vi "Experiment header-Save_Load config file data-retd.vi"(7 "Header file type":T7, 8 "error in (no error)":errorcluster, 9 "All header parameters in":T1={"Imaging Protocol"=enum."AOL Z-Stack", "Number of POI"=0, "Number of Miniscans"=0, "Number of Trials"=0, "Number of Cycles "=0, "# Averaged Frames"=0, "Laser power (%)"=0, "Pockels"=0.0, "Acquisition Length (sec)"=0.0, "Fill time (us)"=0.0, "POI Dwell time (us)"=0.0, "Miniscan Dwell time per pixel (us)"=0.0, "PMT 1"=0.0, "PMT 2"=0.0, "Back Apperture"=0.0, "Zoom"=0.0, "Frame Size"=200, "Center Frequency"=0.0, "Field of View"=0.0, "DwellTime (us)"=0.0, "Wavelength (nm)"=0.0, "AOL Z"=0.0, "AOL Mode"=enum."Raster", "GridXY"=0.0, "GridZ"=0.0, "TriggerDelay (sec)"=0.0, "Number of Pixels in Miniscan"=0, "Experiment folder path"=path "", "X centre"=0.0, "Y centre"=0.0, "Angle (degrees)"=0.0, "Plane Mode"=0, "Software version"=0.0, "Objective"="Olympus  20X", "MotorZ Calibration"=0, "Pockels Calibration"=0, "Threshold"=[], "Video length (sec)"=0.0, "Frame rate (fps)"=0, "Rectangle ROI length (pixels)"=0, "Rectangle ROI height (pixels)"=0} {"Pockels" format="%#.6g"; "Software version" format="%#.6g"; "Plane Mode" items=["XY Plane", "XZ Plane", "YZ Plane", "arbitraryplane"]; "Angle (degrees)" format="%#.6g"; "Frame Size" items=["100X100"=100, "128X128"=128, "200X200"=200, "256X256"=256, "512X512"=512, "1024x1024"=1024, "2048x2048"=2048]; "Back Apperture" format="%#.6g"; "PMT 2" format="%#.6g"; "PMT 1" format="%#.6g"; "Miniscan Dwell time per pixel (us)" format="%#.6g"; "Zoom" format="%#.6g"; "POI Dwell time (us)" format="%#.6g"; "Acquisition Length (sec)" format="%#.6g"; "Fill time (us)" format="%#.6g"}, 10 "Function":T8, 11 "Experiment data folder path":path) -> (0 "error out":errorcluster, 1 "All header parameters out":T1={"Imaging Protocol"=enum."AOL Z-Stack", "Number of POI"=0, "Number of Miniscans"=0, "Number of Trials"=0, "Number of Cycles "=0, "# Averaged Frames"=0, "Laser power (%)"=0, "Pockels"=0.0, "Acquisition Length (sec)"=0.0, "Fill time (us)"=0.0, "POI Dwell time (us)"=0.0, "Miniscan Dwell time per pixel (us)"=0.0, "PMT 1"=0.0, "PMT 2"=0.0, "Back Apperture"=0.0, "Zoom"=0.0, "Frame Size"=200, "Center Frequency"=0.0, "Field of View"=0.0, "DwellTime (us)"=0.0, "Wavelength (nm)"=0.0, "AOL Z"=0.0, "AOL Mode"=enum."Raster", "GridXY"=0.0, "GridZ"=0.0, "TriggerDelay (sec)"=0.0, "Number of Pixels in Miniscan"=0, "Experiment folder path"=path "", "X centre"=0.0, "Y centre"=0.0, "Angle (degrees)"=0.0, "Plane Mode"=0, "Software version"=0.0, "Objective"="Olympus  20X", "MotorZ Calibration"=0, "Pockels Calibration"=0, "Threshold"=[], "Video length (sec)"=0.0, "Frame rate (fps)"=0, "Rectangle ROI length (pixels)"=0, "Rectangle ROI height (pixels)"=0} {"Pockels" format="%#.6g"; "Software version" format="%#.6g"; "Plane Mode" items=["XY Plane", "XZ Plane", "YZ Plane", "arbitraryplane"]; "Angle (degrees)" format="%#.6g"; "Frame Size" items=["100X100"=100, "128X128"=128, "200X200"=200, "256X256"=256, "512X512"=512, "1024x1024"=1024, "2048x2048"=2048]; "Back Apperture" format="%#.6g"; "PMT 2" format="%#.6g"; "PMT 1" format="%#.6g"; "Miniscan Dwell time per pixel (us)" format="%#.6g"; "Zoom" format="%#.6g"; "POI Dwell time (us)" format="%#.6g"; "Acquisition Length (sec)" format="%#.6g"; "Fill time (us)" format="%#.6g"})   [LabVIEW 2017]
doc: "This self-contained module handles all header files save/write operations.\nIt can generate a number of different header files containing different parameters.\nEach different type of header file has its own type defined cluster of parameters.\nThe functionality is fully self-scalable such as when new parameters are added or parameters are deleted or renamed in the typedef clusters this is all handled automatically without the need for further updates to this module."
uses:
  Typedefs/Header parameters cluster-ALL-retd.ctl
  Typedefs/Imaging Protocols enum.ctl
  Typedefs/Frame Size.ctl
  Typedefs/AOL modes.ctl
  Typedefs/Plane Mode.ctl
  Typedefs/Objective selector control enum.ctl
  Typedefs/Save-Load-Save as-Load last enum.ctl
  Typedefs/Header file type enum.ctl
  <vilib>/Utility/config.llb/Read Key (Double).vi
  <vilib>/Utility/config.llb/Write Key (Double).vi
  <vilib>/Utility/config.llb/NI_LVConfig.lvlib
panel:
  # "Actual FOV ------>\n(not norm FOFV)"
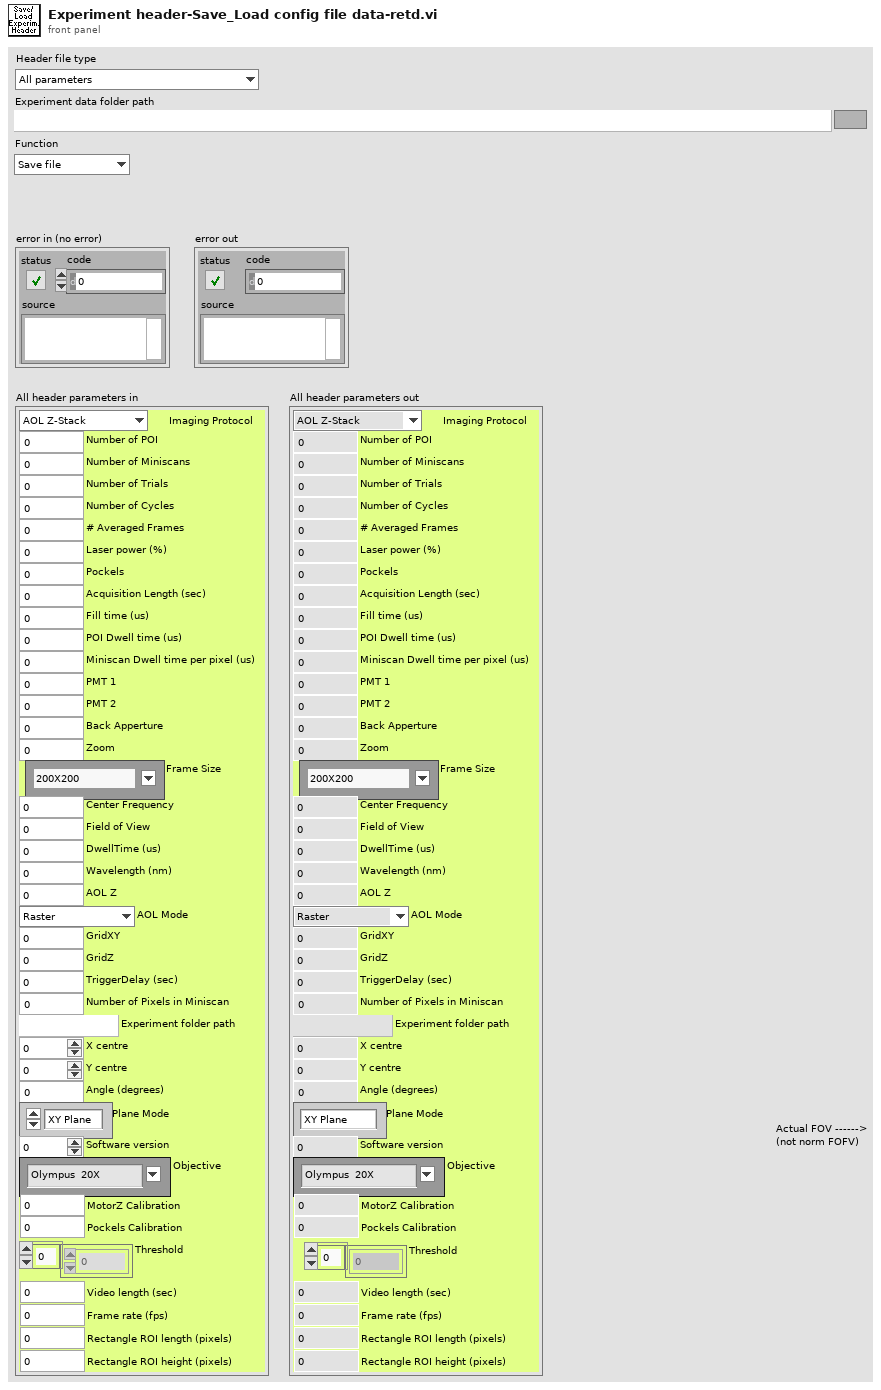
[diagram p1: front panel]
types:
  T1 = typedef "Header parameters cluster-ALL-retd.ctl" = cluster{"Imaging Protocol":T2, "Number of POI":u16, "Number of Miniscans":u16, "Number of Trials":u16, "Number of Cycles ":u64, "# Averaged Frames":u16, "Laser power (%)":u8, "Pockels":dbl, "Acquisition Length (sec)":dbl, "Fill time (us)":dbl, "POI Dwell time (us)":dbl, "Miniscan Dwell time per pixel (us)":dbl, "PMT 1":dbl, "PMT 2":dbl, "Back Apperture":dbl, "Zoom":dbl, "Frame Size":T3, "Center Frequency":dbl, "Field of View":dbl, "DwellTime (us)":dbl, "Wavelength (nm)":dbl, "AOL Z":dbl, "AOL Mode":T4, "GridXY":dbl, "GridZ":dbl, "TriggerDelay (sec)":dbl, "Number of Pixels in Miniscan":u16, "Experiment folder path":path, "X centre":dbl, "Y centre":dbl, "Angle (degrees)":dbl, "Plane Mode":T5, "Software version":dbl, "Objective":T6, "MotorZ Calibration":u32, "Pockels Calibration":u32, "Threshold":u16[], "Video length (sec)":dbl, "Frame rate (fps)":u8, "Rectangle ROI length (pixels)":u16, "Rectangle ROI height (pixels)":u16}
  T2 = typedef "Imaging Protocols enum.ctl" = enum16{"AOL Z-Stack", "Motor Z Stack", "Functional Acquisition", "Single Plane Acquisition", "Volume Acquisition", "Live Imaging", "Live Plane Imaging", "Live Volume Imaging"}
  T3 = typedef "Frame Size.ctl" = u16
  T4 = typedef "AOL modes.ctl" = enum16{"Raster", "Structural", "Pointing", "Mini Scan", "Alignment"}
  T5 = typedef "Plane Mode.ctl" = u16
  T6 = typedef "Objective selector control enum.ctl" = string
  T7 = typedef "Header file type enum.ctl" = enum16{"All parameters", "Login", "Global Parameters", "Imaging Modes", "Time Series", "Motor Zstack", "AOL Zstack", "Functional Imaging", "Movement Correction", "Calibration Setup", "Statistics", "Biology Information"}
  T8 = typedef "Save-Load-Save as-Load last enum.ctl" = enum16{"Save file", "Save file as", "Load file", "Load last file"}
  T9 = typedef "Fixed strings.ctl" = cluster{"ROI file name":string, "Normalised ROI file name":string, "Zplane Pockels values file name":string, "Functional data folder name":string, "Experiment Header file name":string, "Z-stack images folder name":string, "Groups setup rel. path":string, "Groups text file rel. path":string, "TDMS files folder name (F.img)":string, "TDMS files folder name (V.acq)":string, "TDMS files folder name (Pl.acq)":string, "Cycle rel times sequence file":string, "Dynamically called VIs folder name":string, "Time Series folder base name":string}
  T10 = typedef "NI_LVConfig.lvlib/Config Data RefNum.ctl" = refnum<k1>
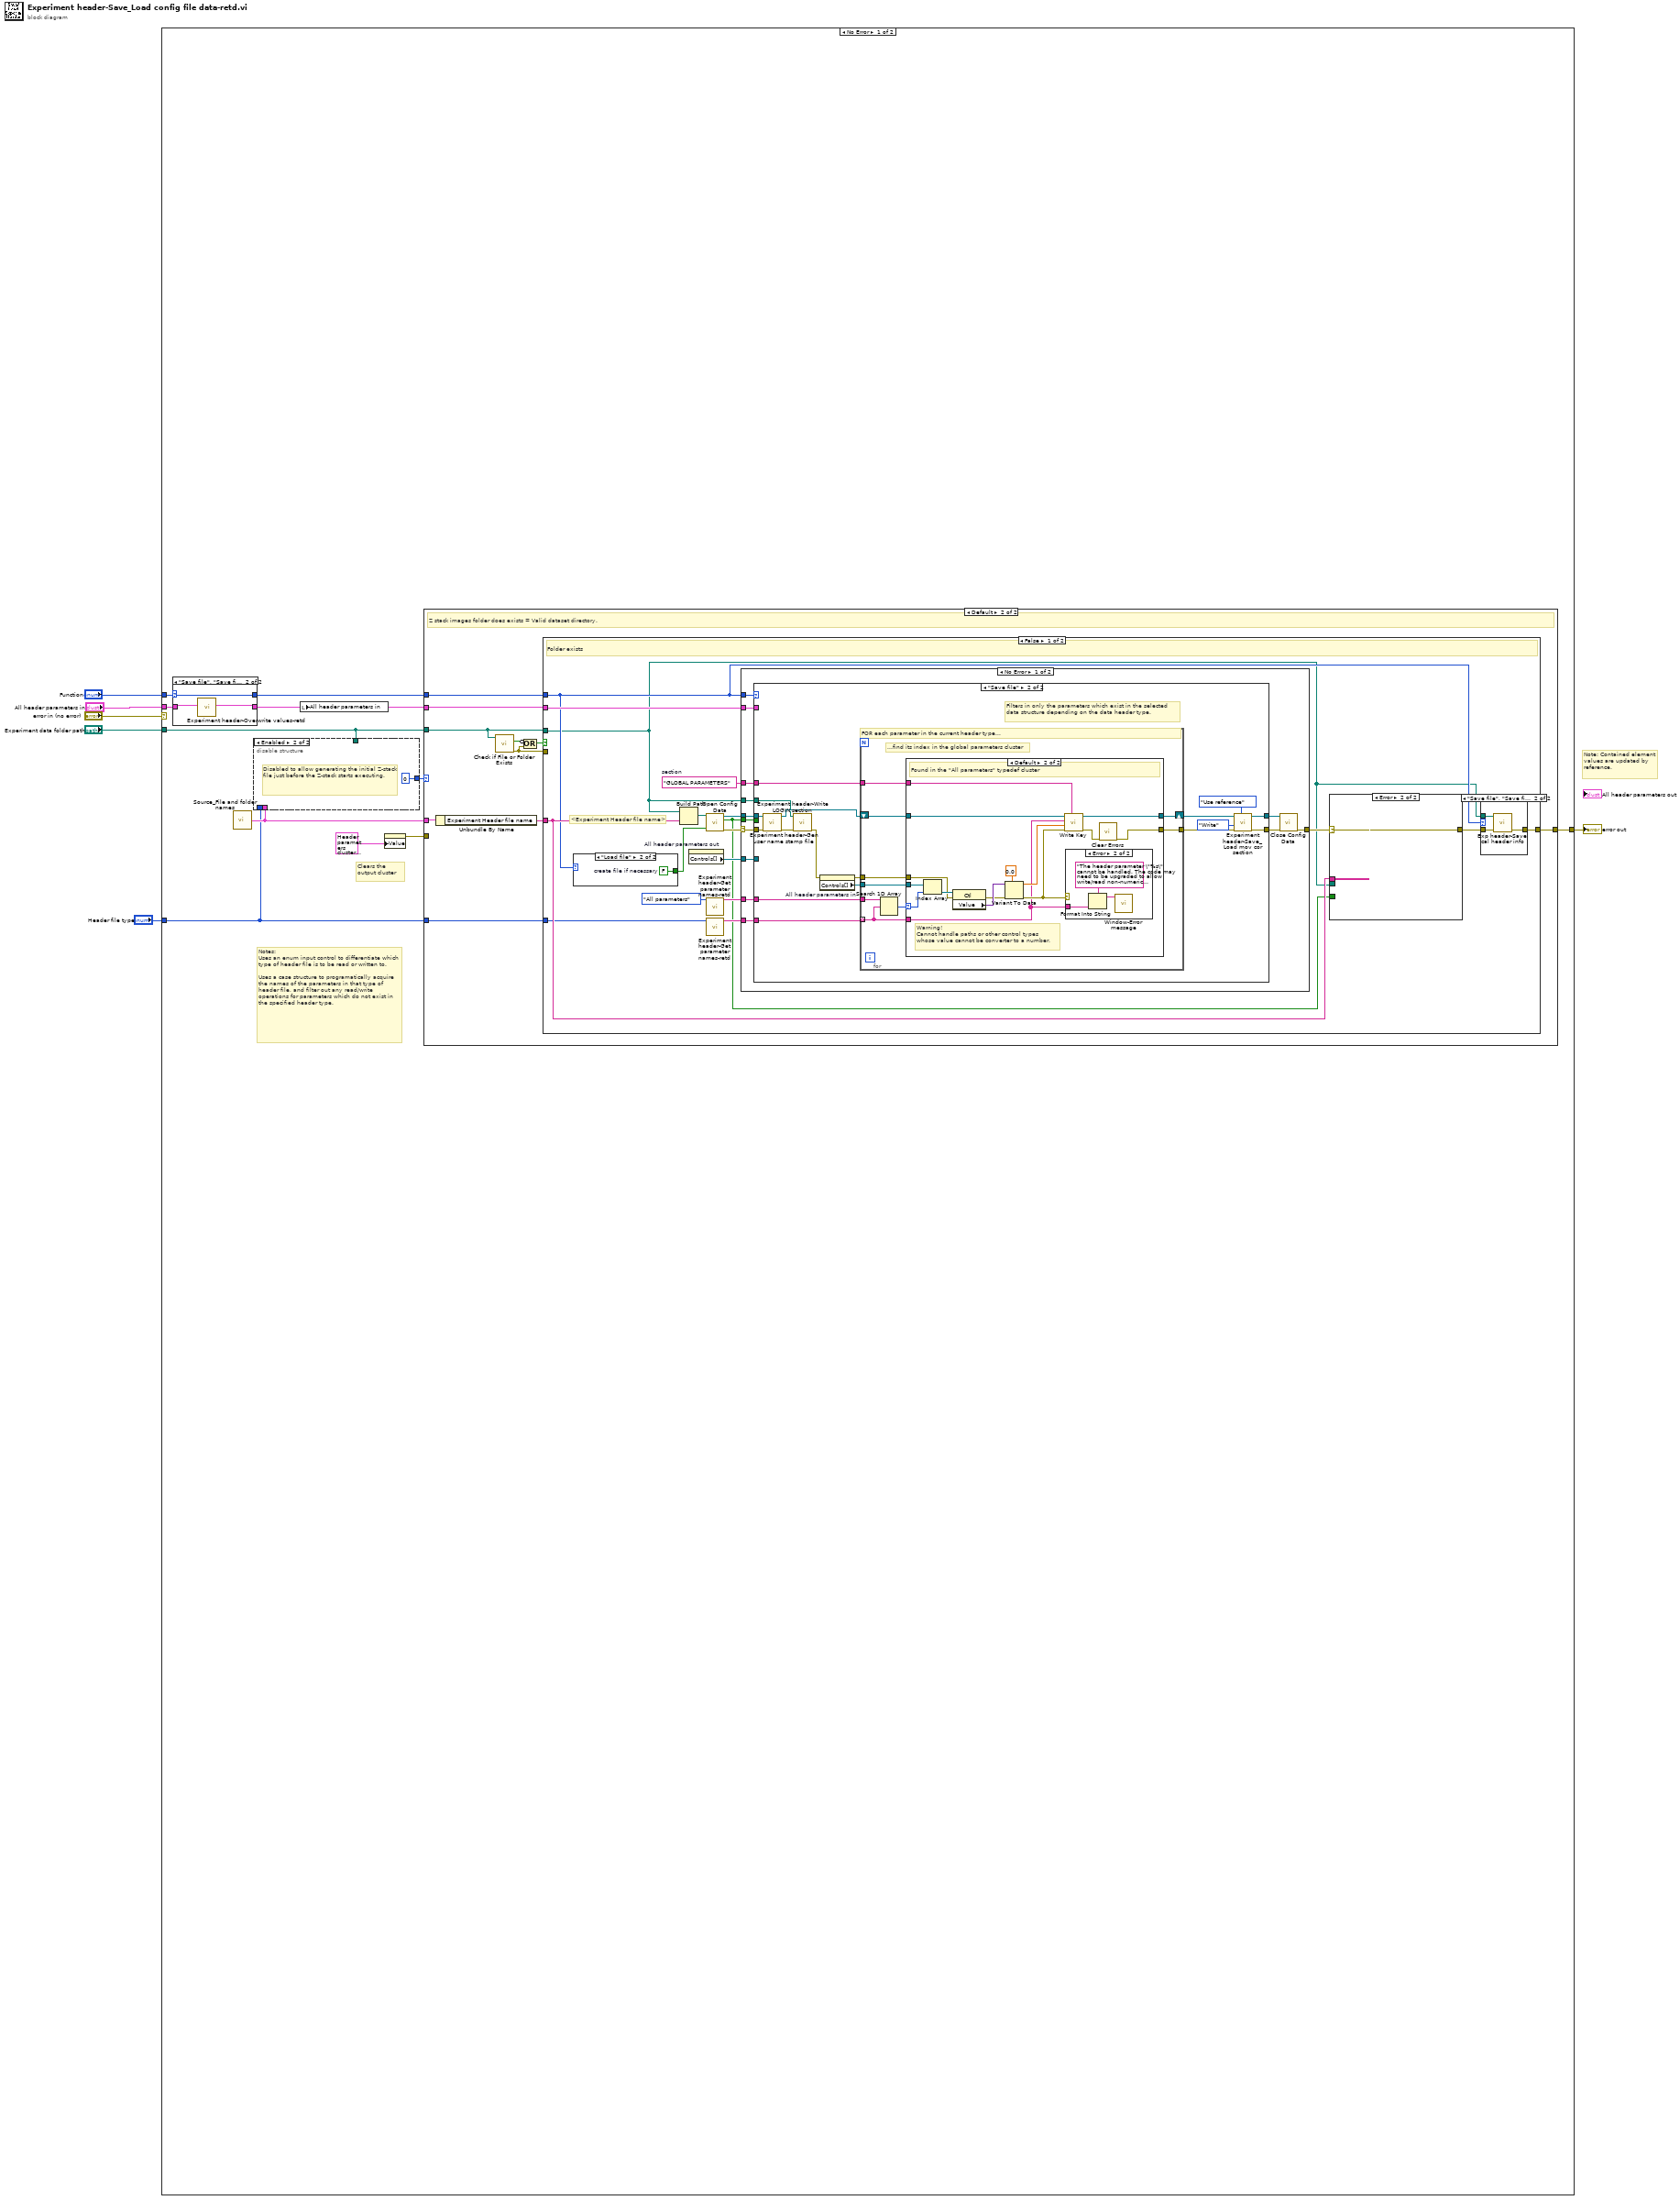
[diagram p0: block diagram]
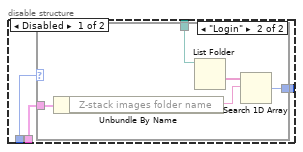
[diagram p3: hidden frame]
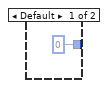
[diagram p4: hidden frame]
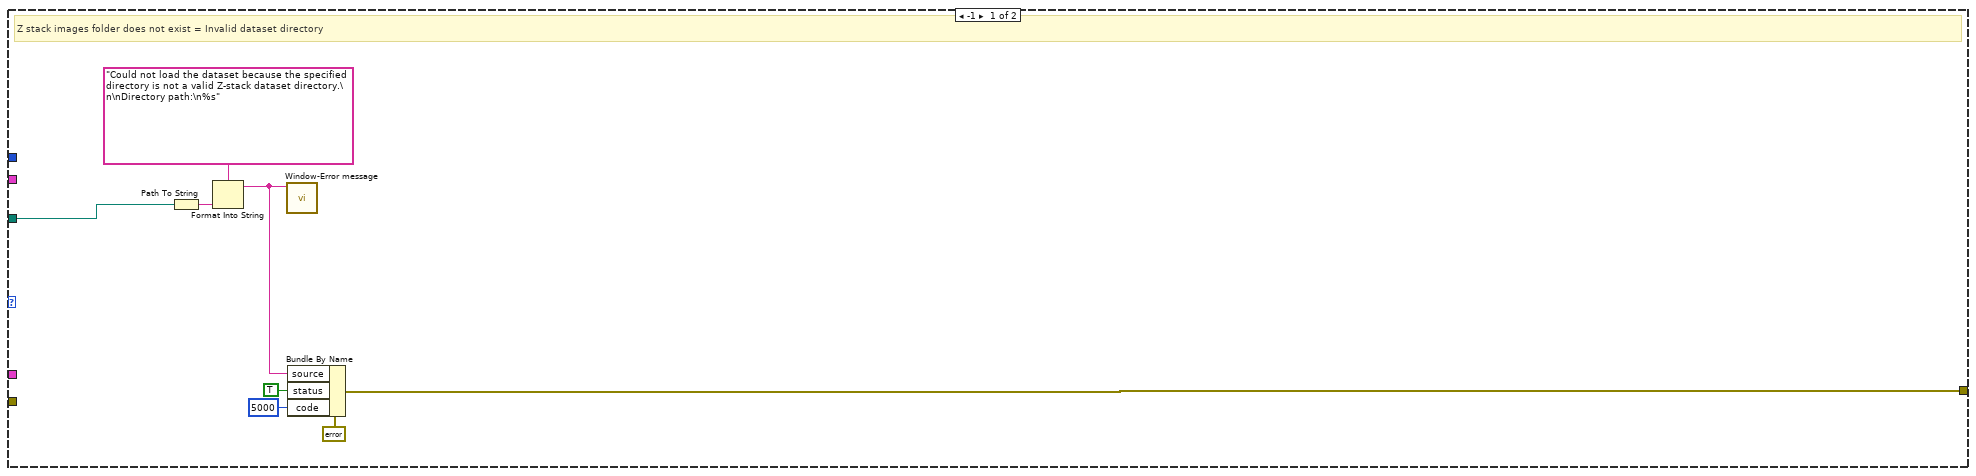
[diagram p5: hidden frame]
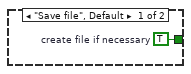
[diagram p7: hidden frame]
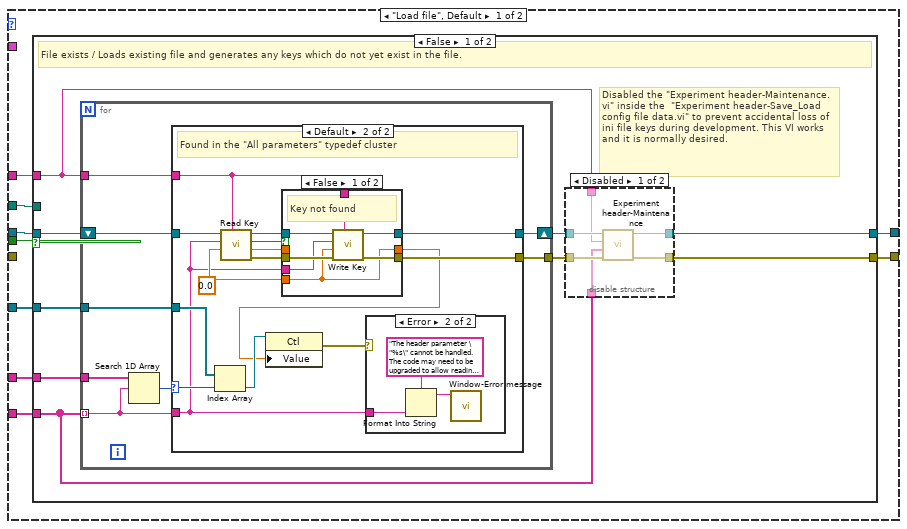
[diagram p8: hidden frame]
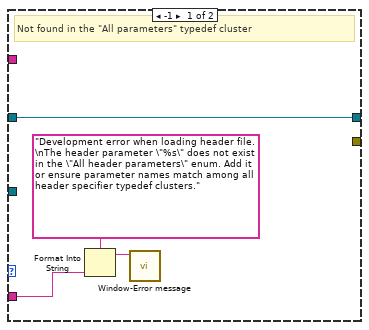
[diagram p10: hidden frame]
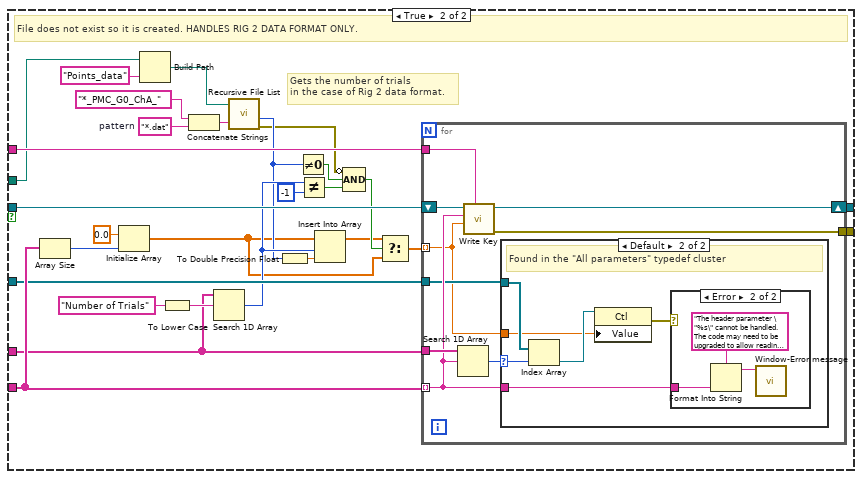
[diagram p13: hidden frame]
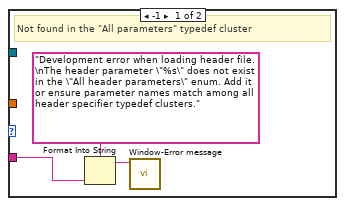
[diagram p14: hidden frame]
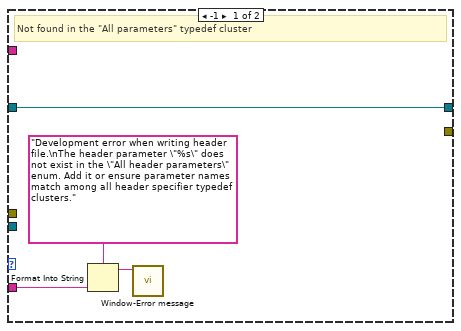
[diagram p16: hidden frame]
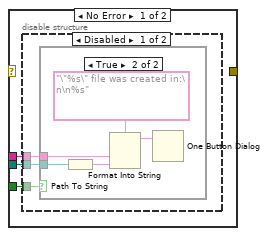
[diagram p19: hidden frame]
diagram:
  # "Note: Contained element values are updated by reference."
  n1 = case shown="No Error" "error in (no error)" {
    selector: "error in (no error)" -> [_ w277]
    tunnel: [w17 w277] -> w6
    tunnel: "Function" -> [w11 _]
    tunnel: "Experiment data folder path" -> [w9 _]
    tunnel: "Header file type" -> [w13 _]
    tunnel: "All header parameters in" -> [w10 _]
    frame No Error {
      # "Clears the output cluster"
      # "Notes:\nUses an enum input control to differentiate which type of header file is to be read or written to.\n\nUses a case structure to programatically acquire the names of the parameters in that type of header file, and filter out any read/write operations for parameters which do not exist in the specified header type."
      n2 = case shown="\"Save file\", \"Save file as\"" w11 {
        selector: w11 -> [w19 w22]
        tunnel: [w18 w20] -> w8
        tunnel: [w19 w22] -> w12
        tunnel: w10 -> [w18 w21]
        frame Default {
        }
        frame "Save file", "Save file as" {
          n3 = call "Experiment header-Overwrite values-retd.vi"("All header parameters in"=w21) -> ("All header parameters (FOV converted to um)"=w20:T1)  [unwired: 9 in, 1 out]
        }
      }
      n4 = call "Source_File and folder names.vi"() -> ("Fixed strings"=w15:T9)  [unwired: 1 in]
      n5 = disable-structure shown="Enabled" {
        disable-tunnel: w9 -> [w26 _]
        disable-tunnel: [w25 0 ("index of element")] -> w16
        disable-tunnel: w15 -> [w24 _]
        disable-tunnel: w13 -> [w23 _]
        frame Disabled {
          n6 = case shown="\"Login\"" w23 {
            tunnel: w26 -> [_ w31]
            tunnel: [0 ("index of element") w30] -> w25
            tunnel: w24 -> [_ w28]
            frame Default {
            }
            frame "Login" {
              n7 = Unbundle By Name(w28) -> ("Z-stack images folder name"=w29:string)
              n8 = List Folder(path=w31) -> (folder names=w32:string[])  [unwired: 3 in, 3 out]
              n9 = Search 1D Array(1D array=w32, element=w29) -> (index of element=w30:i32)  [unwired: 1 in]
            }
          }
        }
        frame Enabled {
          # "Disabled to allow generating the initial Z-stack file just before the Z-stack starts executing."
        }
      }
      n10 = local write "All header parameters in"(w8) -> ()
      n11 = property on="All header parameters out" class="Clust (strict)"("Value"=T1 {"Imaging Protocol"=enum."AOL Z-Stack", "Number of POI"=0, "Number of Miniscans"=0, "Number of Trials"=0, "Number of Cycles "=0, "# Averaged Frames"=0, "Laser power (%)"=0, "Pockels"=0.0, "Acquisition Length (sec)"=0.0, "Fill time (us)"=0.0, "POI Dwell time (us)"=0.0, "Miniscan Dwell time per pixel (us)"=0.0, "PMT 1"=0.0, "PMT 2"=0.0, "Back Apperture"=0.0, "Zoom"=0.0, "Frame Size"=200, "Center Frequency"=0.0, "Field of View"=0.0, "DwellTime (us)"=0.0, "Wavelength (nm)"=0.0, "AOL Z"=0.0, "AOL Mode"=enum."Raster", "GridXY"=0.0, "GridZ"=0.0, "TriggerDelay (sec)"=0.0, "Number of Pixels in Miniscan"=0, "Experiment folder path"=path "", "X centre"=0.0, "Y centre"=0.0, "Angle (degrees)"=0.0, "Plane Mode"=0, "Software version"=0.0, "Objective"="Olympus  20X", "MotorZ Calibration"=0, "Pockels Calibration"=0, "Threshold"=[], "Video length (sec)"=0.0, "Frame rate (fps)"=0, "Rectangle ROI length (pixels)"=0, "Rectangle ROI height (pixels)"=0} ("All header parameters / Header module interface cluster")) -> (error out=w14:errorcluster)  [unwired: 2 in, 1 out]
      n12 = case shown="Default" w16 {
        tunnel: [w34 w51] -> w17
        tunnel: w12 -> [_ w47]
        tunnel: w8 -> [_ w46]
        tunnel: w9 -> [w39 w45]
        tunnel: w15 -> [_ w43]
        tunnel: w13 -> [_ w42]
        tunnel: w14 -> [_ _]
        frame -1 {
          # "Z stack images folder does not exist = Invalid dataset directory"
          n13 = Path To String(path=w39) -> (string=w41:string)
          n14 = Format Into String(format string="Could not load the dataset because the specified directory is not a valid Z-stack dataset directory.\n\nDirectory path:\n%s" ("message"), w41) -> (resulting string=w35:string)  [unwired: 2 in, 1 out]
          n15 = call "Window-Error message.vi"("Message"=w35) -> ()  [unwired: 10 in, 1 out]
          n16 = Bundle By Name(cluster=errorcluster {"status"=FALSE, "code"=0, "source"=""} ("error out"), "source"=w35, "status"=TRUE, "code"=5000) -> (w34:errorcluster)
        }
        frame Default {
          # "Z stack images folder does exists = Valid dataset directory."
          n17 = Unbundle By Name(w43) -> ("Experiment Header file name"=w44:string)
          n18 = call <vilib>:"Check if File or Folder Exists.vi"("path"=w45) -> ("error out"=w48:errorcluster, "file or folder exists?"=w50:bool)  [unwired: 8 in, 1 out]
          n19 = Compound Arithmetic op=OR(invert w50, w48) -> (w49:bool)
          n20 = case shown="False" w49 {
            tunnel: [w55 w266] -> w51
            tunnel: w44 -> [w64 _]
            tunnel: w45 -> [w52 w267]
            tunnel: w48 -> [_ w265]
            tunnel: w47 -> [w53 _]
            tunnel: w46 -> [w69 _]
            tunnel: w42 -> [w63 _]
            frame False {
              w58 = "GLOBAL PARAMETERS"  # section
              # "<Experiment Header file name>"
              # "Folder exists"
              n21 = case shown="\"Load file\"" w53 {
                tunnel: [w74 w75] -> w56
                frame "Save file", Default {
                  w74 = TRUE  # create file if necessary
                }
                frame "Load file" {
                  w75 = FALSE  # create file if necessary
                }
              }
              n22 = Build Path(base path=w52, name or relative path=w64) -> (appended path=w68:path)
              n23 = property on="All header parameters out" class="Clust (strict)"() -> ("Controls[]"=w60:refnum<vi>[])  [unwired: 2 in, 2 out]
              n24 = call <vilib>:"Open Config Data.vi"("create file if necessary (T)"=w56, "configuration file path"=w68) -> ("error out"=w61:errorcluster, "file created?"=w59:bool, "refnum"=w67:T10)  [unwired: 7 in]
              n25 = call "Experiment header-Get parameter names-retd.vi"("Header file type"=Header_file_type_enum."All parameters") -> ("Parameter names"=w62:string[])  [unwired: 9 in, 1 out]
              n26 = call "Experiment header-Get parameter names-retd.vi"("Header file type"=w63) -> ("Parameter names"=w65:string[])  [unwired: 9 in, 1 out]
              n27 = case shown="No Error" w61 {
                selector: w61 -> [w76 w252]
                tunnel: w58 -> [w88 _]
                tunnel: w53 -> [w87 _]
                tunnel: w69 -> [w86 _]
                tunnel: w67 -> [w85 _]
                tunnel: [w82 w252] -> w66
                tunnel: w65 -> [w81 _]
                tunnel: w52 -> [w80 _]
                tunnel: w59 -> [w79 _]
                tunnel: w62 -> [w78 _]
                tunnel: w60 -> [w77 _]
                frame No Error {
                  n28 = case shown="\"Save file\"" w87 {
                    tunnel: [w92 w214] -> w83
                    tunnel: w88 -> [w97 w220]
                    tunnel: w86 -> [_ _]
                    tunnel: w81 -> [w96 w219]
                    tunnel: w79 -> [w94 _]
                    tunnel: w85 -> [w95 w218]
                    tunnel: [w93 w212] -> w84
                    tunnel: w80 -> [w91 w206]
                    tunnel: w78 -> [w90 w217]
                    tunnel: w77 -> [w89 _]
                    tunnel: w76 -> [_ w208]
                    frame "Load file", Default {
                      n29 = case shown="False" w94 {
                        tunnel: w95 -> [w106 w182]
                        tunnel: w97 -> [w99 w181]
                        tunnel: w96 -> [w100 w170]
                        tunnel: [w103 w180] -> w93
                        tunnel: [w102 w179] -> w92
                        tunnel: w91 -> [_ w169]
                        tunnel: w90 -> [w101 w166]
                        tunnel: w89 -> [w98 w165]
                        frame False {
                          # "Disabled the \"Experiment header-Maintenance.vi\" inside the  \"Experiment header-Save_Load config file data.vi\" to prevent accidental loss of ini file keys during development. This VI works and it is normally desired."
                          # "File exists / Loads existing file and generates any keys which do not yet exist in the file."
                          n30 = for {
                            shift-right: [w121] -> w105
                            shift-left: w106 -> [w122]
                            tunnel: w99 -> [w120]
                            tunnel: [w119] -> w104
                            tunnel: w100 -> [w117] mode=indexing
                            tunnel: w101 -> [w118]
                            tunnel: w98 -> [w115]
                            n31 = Search 1D Array(1D array=w118, element=w117) -> (index of element=w116:i32)  [unwired: 1 in]
                            n32 = case shown="Default" w116 {
                              selector: w116 -> [_ w131]
                              tunnel: w122 -> [w124 w141]
                              tunnel: [w124 w139] -> w121
                              tunnel: w120 -> [_ w137]
                              tunnel: [_ w135] -> w119
                              tunnel: w117 -> [w123 w127]
                              tunnel: w115 -> [_ w130]
                              frame -1 {
                                # "Not found in the \"All parameters\" typedef cluster"
                                n33 = Format Into String(format string="Development error when loading header file.\nThe header parameter \"%s\" does not exist in the \"All header parameters\" enum. Add it or ensure parameter names match among all header specifier typedef clusters.", w123) -> (resulting string=w125:string)  [unwired: 2 in, 1 out]
                                n34 = call "Window-Error message.vi"("Message"=w125) -> ()  [unwired: 10 in, 1 out]
                              }
                              frame Default {
                                w133 = 0.0 ("default value")
                                # "Found in the \"All parameters\" typedef cluster"
                                n35 = Index Array(array=w130, index=w131) -> (element=w132:refnum<vi>)
                                n36 = call-poly <vilib>:"Read Key.vi"("section"=w137, "default value"=w133, "key"=w127, "refnum"=w141) -> ("error out"=w136:errorcluster, "value"=w138:dbl, "found?"=w134:bool, "refnum out"=w140:T10)  [unwired: 4 in]
                                n37 = case shown="False" w134 {
                                tunnel: w140 -> [w151 w154]
                                tunnel: [w150 w154] -> w139
                                tunnel: w138 -> [_ w153]
                                tunnel: [w146 w153] -> w129
                                tunnel: w137 -> [w149 _]
                                tunnel: w133 -> [w146 _]
                                tunnel: w136 -> [w148 w152]
                                tunnel: [w147 w152] -> w135
                                tunnel: w127 -> [w145 _]
                                frame False {
                                # "Key not found"
                                n38 = call-poly <vilib>:"Write Key.vi"("section"=w149, "error in (no error)"=w148, "value"=w146, "key"=w145, "refnum"=w151) -> ("error out"=w147:errorcluster, "refnum out"=w150:T10)  [unwired: 4 in, 1 out]
                                }
                                frame True {
                                # "Key found"
                                }
                                }
                                n39 = property class="Ctl"(reference=w132, "Value"=w129) -> (error out=w128:errorcluster)  [unwired: 1 in, 1 out]
                                n40 = case shown="Error" w128 {
                                tunnel: w127 -> [_ w143]
                                frame No Error {
                                }
                                frame Error {
                                n41 = Format Into String(format string="The header parameter \"%s\" cannot be handled. The code may need to be upgraded to allow reading non-numeric parameter values from the header file.", w143) -> (resulting string=w144:string)  [unwired: 2 in, 1 out]
                                n42 = call "Window-Error message.vi"("Message"=w144) -> ()  [unwired: 10 in, 1 out]
                                }
                                }
                              }
                            }
                          }
                          n43 = disable-structure shown="Disabled" {
                            disable-tunnel: w105 -> [w112 w114]
                            disable-tunnel: w104 -> [w111 w113]
                            disable-tunnel: [w110 w114] -> w103
                            disable-tunnel: [w109 w113] -> w102
                            disable-tunnel: w100 -> [w108 _]
                            disable-tunnel: w99 -> [w107 _]
                            frame Disabled {
                              n44 = call "Experiment header-Maintenance.vi"("error in (no error)"=w111, "<Valid parameter names>"=w108, "section"=w107, "Experiment header file ref in"=w112) -> ("error out"=w109:errorcluster, "Experiment header file ref"=w110:T10)  [unwired: 6 in]
                            }
                            frame Enabled {
                            }
                          }
                        }
                        frame True {
                          w175 = "*.dat"  # pattern
                          # "Gets the number of trials\nin the case of Rig 2 data format."
                          # "File does not exist so it is created. HANDLES RIG 2 DATA FORMAT ONLY."
                          n45 = Array Size(array=w170) -> (size(s)=w173:i32)
                          n46 = Initialize Array(0.0, w173) -> (w157:dbl[])
                          n47 = Build Path(base path=w169, name or relative path="Points_data") -> (appended path=w174:path)
                          n48 = To Lower Case(string="Number of Trials" ("element")) -> (all lower case string=w167:string)
                          n49 = Concatenate Strings("*_PMC_G0_ChA_" ("string"), w175) -> (w176:string)
                          n50 = Search 1D Array(1D array=w166, element=w167) -> (index of element=w164:i32)  [unwired: 1 in]
                          n51 = call <vilib>:"Recursive File List.vi"("pattern"=w176, "Folder Path"=w174) -> ("error out"=w155:errorcluster, "Number of Files"=w162:i32)  [unwired: 5 in, 3 out]
                          n52 = To Double Precision Float(number=w162) -> (double precision float=w171:dbl)
                          n53 = Not Equal To 0?(x=w162) -> (x != 0?=w161:bool)
                          n54 = Not Equal?(x=w164, y=-1) -> (x != y?=w160:bool)
                          n55 = Insert Into Array(array=w157, index=w164, new element=w171) -> (w158:dbl[])
                          n56 = Compound Arithmetic op=AND(invert w155, w161, w160) -> (w159:bool)
                          n57 = Select(t=w158, s=w159, f=w157) -> (s? t:f=w156:dbl[])
                          n58 = for {
                            shift-right: [w190] -> w180
                            shift-left: w182 -> [w191]
                            tunnel: w181 -> [w189]
                            tunnel: [w188] -> w179
                            tunnel: w170 -> [w185] mode=indexing
                            tunnel: w156 -> [w183] mode=indexing
                            tunnel: w166 -> [w186]
                            tunnel: w165 -> [w184]
                            n59 = Search 1D Array(1D array=w186, element=w185) -> (index of element=w187:i32)  [unwired: 1 in]
                            n60 = call-poly <vilib>:"Write Key.vi"("section"=w189, "value"=w183, "key"=w185, "refnum"=w191) -> ("error out"=w188:errorcluster, "refnum out"=w190:T10)  [unwired: 5 in, 1 out]
                            n61 = case shown="Default" w187 {
                              selector: w187 -> [_ w199]
                              tunnel: w185 -> [w192 w196]
                              tunnel: w184 -> [_ w198]
                              tunnel: w183 -> [_ w195]
                              frame -1 {
                                # "Not found in the \"All parameters\" typedef cluster"
                                n62 = Format Into String(format string="Development error when loading header file.\nThe header parameter \"%s\" does not exist in the \"All header parameters\" enum. Add it or ensure parameter names match among all header specifier typedef clusters.", w192) -> (resulting string=w193:string)  [unwired: 2 in, 1 out]
                                n63 = call "Window-Error message.vi"("Message"=w193) -> ()  [unwired: 10 in, 1 out]
                              }
                              frame Default {
                                # "Found in the \"All parameters\" typedef cluster"
                                n64 = Index Array(array=w198, index=w199) -> (element=w200:refnum<vi>)
                                n65 = property class="Ctl"(reference=w200, "Value"=w195) -> (error out=w197:errorcluster)  [unwired: 1 in, 1 out]
                                n66 = case shown="Error" w197 {
                                tunnel: w196 -> [_ w202]
                                frame No Error {
                                }
                                frame Error {
                                n67 = Format Into String(format string="The header parameter \"%s\" cannot be handled. The code may need to be upgraded to allow reading non-numeric parameter values from the header file.", w202) -> (resulting string=w203:string)  [unwired: 2 in, 1 out]
                                n68 = call "Window-Error message.vi"("Message"=w203) -> ()  [unwired: 10 in, 1 out]
                                }
                                }
                              }
                            }
                          }
                        }
                      }
                    }
                    frame "Save file" {
                      # "Filters in only the parameters which exist in the selected data structure depending on the data header type."
                      n69 = call "Experiment header-Write LOGIN section.vi"("error in (no error)"=w208, "Experiment header file ref"=w218) -> ("error out"=w205:errorcluster, "Experiment header file ref"=w209:T10)  [unwired: 8 in]
                      n70 = call "Experiment header-Gen user name stamp file.vi"("error in (no error)"=w205, "Experiment data folder path"=w206) -> ("error out"=w204:errorcluster)  [unwired: 9 in]
                      n71 = property on="All header parameters in" class="Clust (strict)"(error in=w204) -> (error out=w207:errorcluster, "Controls[]"=w216:refnum<vi>[])  [unwired: 1 in, 1 out]
                      n72 = for {
                        shift-right: [w228] -> w215
                        shift-left: w209 -> [w229]
                        tunnel: w220 -> [w227]
                        tunnel: w219 -> [w224] mode=indexing
                        tunnel: w217 -> [w225]
                        tunnel: w216 -> [w223]
                        tunnel: [w222] -> w213
                        tunnel: w207 -> [w221]
                        # "...find its index in the global parameters cluster"
                        # "FOR each parameter in the current header type..."
                        n73 = Search 1D Array(1D array=w225, element=w224) -> (index of element=w226:i32)  [unwired: 1 in]
                        n74 = case shown="Default" w226 {
                          selector: w226 -> [_ w245]
                          tunnel: w229 -> [w233 w248]
                          tunnel: [w233 w247] -> w228
                          tunnel: w227 -> [_ w246]
                          tunnel: w224 -> [w232 w237]
                          tunnel: w223 -> [_ w241]
                          tunnel: [_ w235] -> w222
                          tunnel: w221 -> [_ w234]
                          frame -1 {
                            # "Not found in the \"All parameters\" typedef cluster"
                            n75 = Format Into String(format string="Development error when writing header file.\nThe header parameter \"%s\" does not exist in the \"All header parameters\" enum. Add it or ensure parameter names match among all header specifier typedef clusters.", w232) -> (resulting string=w231:string)  [unwired: 2 in, 1 out]
                            n76 = call "Window-Error message.vi"("Message"=w231) -> ()  [unwired: 10 in, 1 out]
                          }
                          frame Default {
                            # "Warning!\nCannot handle paths or other control types \nwhose value cannot be converter to a number."
                            # "Found in the \"All parameters\" typedef cluster"
                            n77 = Index Array(array=w241, index=w245) -> (element=w244:refnum<vi>)
                            n78 = property class="Ctl"(reference=w244, error in=w234) -> (error out=w239:errorcluster, "Value"=w243:variant)  [unwired: 1 out]
                            n79 = Variant To Data(error in=w239, type=0.0, Variant=w243) -> (data=w240:dbl, error out=w238:errorcluster)
                            n80 = call-poly <vilib>:"Write Key.vi"("section"=w246, "error in (no error)"=w238, "value"=w240, "key"=w237, "refnum"=w248) -> ("error out"=w236:errorcluster, "refnum out"=w247:T10)  [unwired: 4 in, 1 out]
                            n81 = case shown="Error" w238 {
                              tunnel: w237 -> [_ w249]
                              frame No Error {
                              }
                              frame Error {
                                n82 = Format Into String(format string="The header parameter \"%s\" cannot be handled. The code may need to be upgraded to allow write/read non-numeric parameter values to the header file.", w249) -> (resulting string=w250:string)  [unwired: 2 in, 1 out]
                                n83 = call "Window-Error message.vi"("Message"=w250) -> ()  [unwired: 10 in, 1 out]
                              }
                            }
                            n84 = call <vilib>:"Clear Errors.vi"("error in (no error)"=w236) -> ("error out"=w235:errorcluster)  [unwired: 5 in, 1 out]
                          }
                        }
                      }
                      n85 = call "Experiment header-Save_Load mov cor section.vi"("Input Mode (ref)"=enum16{"Use reference", "Use folder path"}."Use reference", "error in (no error)"=w213, "Function"=enum16{"Write", "Read"}."Write", "Exp header file ref in"=w215) -> ("error out"=w214:errorcluster, "Exp header file ref"=w212:T10)  [unwired: 5 in, 1 out]
                    }
                  }
                  n86 = call <vilib>:"Close Config Data.vi"("error in (no error)"=w83, "refnum"=w84) -> ("error out"=w82:errorcluster)  [unwired: 8 in, 1 out]
                }
                frame Error {
                }
              }
              n87 = case shown="Error" w66 {
                selector: w66 -> [_ w264]
                tunnel: [_ w264] -> w54
                tunnel: w59 -> [w255 _]
                tunnel: w52 -> [w254 _]
                tunnel: w64 -> [w253 _]
                frame No Error {
                  n88 = disable-structure shown="Disabled" {
                    disable-tunnel: w255 -> [w258 _]
                    disable-tunnel: w254 -> [w257 _]
                    disable-tunnel: w253 -> [w256 _]
                    frame Disabled {
                      n89 = case shown="True" w258 {
                        tunnel: w257 -> [_ w261]
                        tunnel: w256 -> [_ w259]
                        frame False {
                        }
                        frame True {
                          n90 = Path To String(path=w261) -> (string=w260:string)
                          n91 = Format Into String(format string="\"%s\" file was created in:\n\n%s" ("message"), w259, w260) -> (resulting string=w262:string)  [unwired: 2 in, 1 out]
                          n92 = One Button Dialog(message=w262) -> ()  [unwired: 1 in, 1 out]
                        }
                      }
                    }
                    frame Enabled {
                    }
                  }
                }
                frame Error {
                }
              }
              n93 = case shown="\"Save file\", \"Save file as\"" w53 {
                tunnel: [w70 w73] -> w55
                tunnel: w54 -> [w70 w72]
                tunnel: w52 -> [_ w71]
                frame Default {
                }
                frame "Save file", "Save file as" {
                  n94 = call "Exp header-Save cal header info.vi"("error in (no error)"=w72, "Experiment folder path"=w71) -> ("error out"=w73:errorcluster)  [unwired: 9 in]
                }
              }
            }
            frame True {
              # "Folder foes not exist! OR Error"
              n95 = case shown="No Error" w265 {
                selector: w265 -> [_ w276]
                tunnel: w267 -> [w273 _]
                tunnel: [w271 w276] -> w266
                frame No Error {
                  n96 = Path To String(path=w273) -> (string=w274:string)
                  n97 = Format Into String(format string="\"Experiment Header.ini\" file could not be accessed because the specified folder path does not exist.\n\nPath:\n%s" ("message"), w274) -> (resulting string=w268:string)  [unwired: 2 in, 1 out]
                  n98 = call "Window-Error message.vi"("Message"=w268) -> ()  [unwired: 10 in, 1 out]
                  n99 = Bundle By Name(cluster=errorcluster {"status"=FALSE, "code"=0, "source"=""} ("error out"), "source"=w268, "status"=TRUE, "code"=5000) -> (w271:errorcluster)
                }
                frame Error {
                }
              }
            }
          }
        }
      }
    }
    frame Error {
    }
  }
  "error out" <- w6
